vi "13-14-高级计算器.vi"() -> ()   [LabVIEW 2025]
panel:
  out "过程显示":string
  in  "清除":bool
  in  "等于":bool
  in  "小数点":bool
  in  "±号":bool
  in  "数字0":bool
  in  "操作/":bool
  in  "操作*":bool
  in  "数字9":bool
  in  "数字8":bool
  in  "数字7":bool
  in  "数字6":bool
  in  "数字5":bool
  in  "数字4":bool
  in  "操作-":bool
  in  "操作+":bool
  in  "数字3":bool
  in  "数字2":bool
  in  "数字1":bool
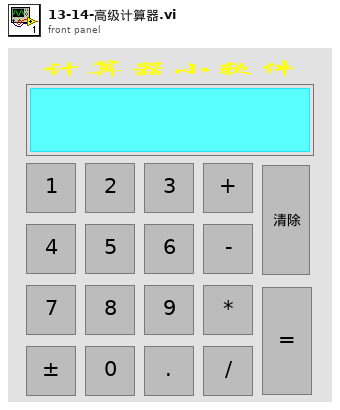
[diagram p1: front panel]
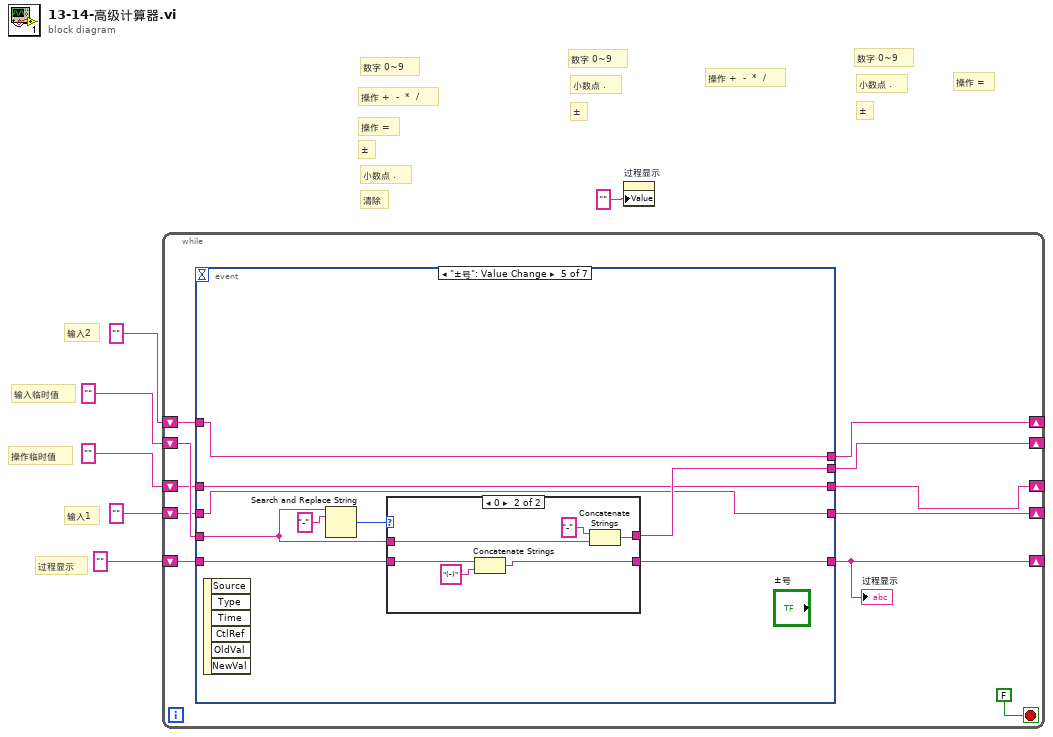
[diagram p0: block diagram]
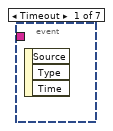
[diagram p2: hidden frame]
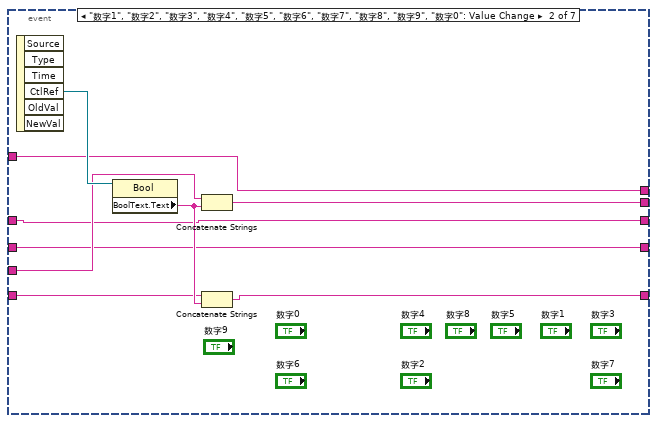
[diagram p3: hidden frame]
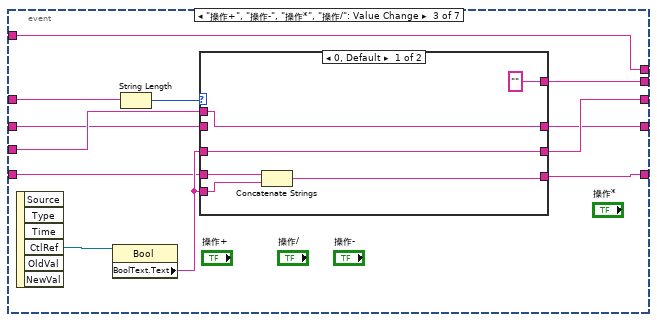
[diagram p4: hidden frame]
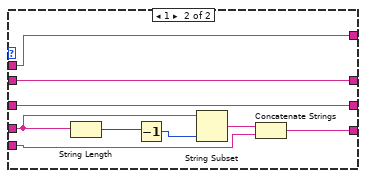
[diagram p5: hidden frame]
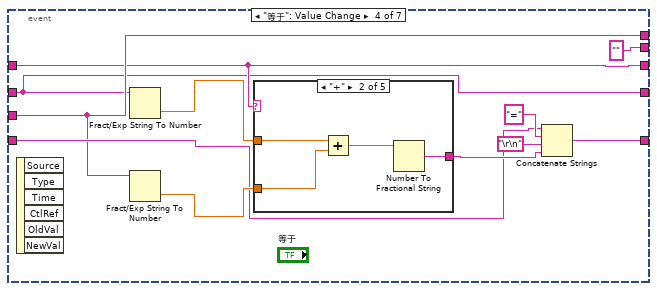
[diagram p6: hidden frame]
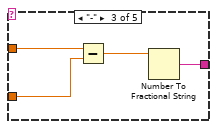
[diagram p8: hidden frame]
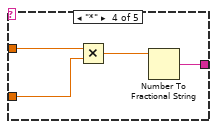
[diagram p9: hidden frame]
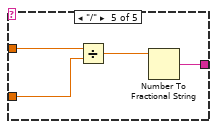
[diagram p10: hidden frame]
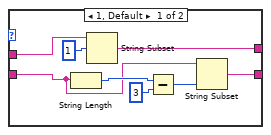
[diagram p11: hidden frame]
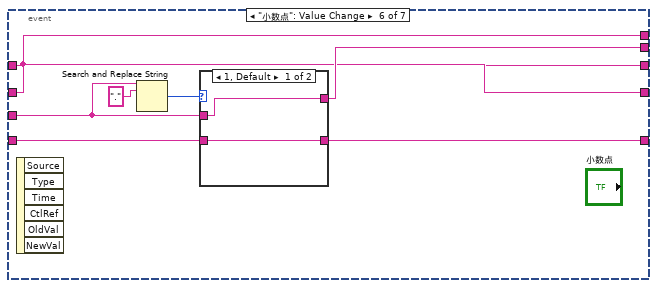
[diagram p12: hidden frame]
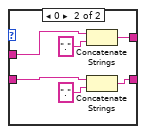
[diagram p13: hidden frame]
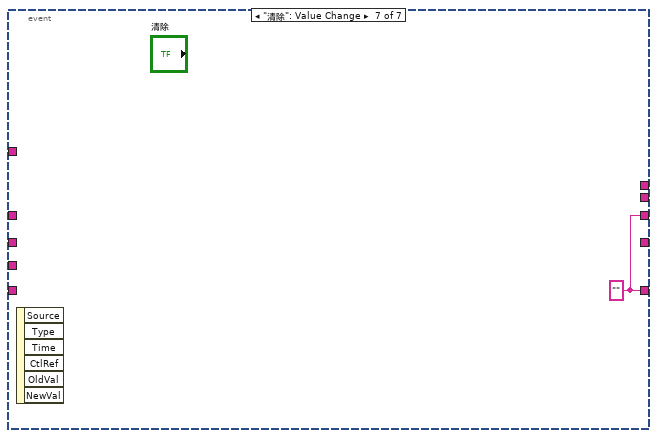
[diagram p14: hidden frame]
diagram:
  # "操作临时值"
  # "过程显示"
  # "输入2"
  # "输入1"
  # "输入临时值"
  # "操作 ="
  # "±"
  # "小数点 ."
  # "数字 0~9"
  # "操作 +  -  *  /"
  # "±"
  # "小数点 ."
  # "数字 0~9"
  # "清除"
  # "小数点 ."
  # "±"
  # "操作 ="
  # "操作 +  -  *  /"
  # "数字 0~9"
  n1 = while {
    shift-right: [w15] -> _
    shift-left: "" ("输入1") -> [w16]
    shift-right: [w11] -> _
    shift-left: "" ("输入1") -> [w10]
    shift-right: [w9] -> _
    shift-left: "" ("输入1") -> [w8]
    shift-right: [w7] -> _
    shift-left: "" ("输入1") -> [w14]
    shift-right: [w12] -> _
    shift-left: "" ("输入1") -> [w13]
    stop <- FALSE stop-if-true
    n2 = event shown="[4] \"±号\": Value Change" {
      selector: _ -> [_ _ _ _ _ _ _]
      dyn-events: _ -> [_ _ _ _ _ _ _]
      timeout: _ -> [_ _ _ _ _ _ _]
      tunnel: w16 -> [_ w24 w32 w56 w85 w109 _]
      tunnel: [_ w23 w30 "" ("输入临时值") w84 w108 _] -> w15
      tunnel: w14 -> [_ w22 w35 w59 w87 w107 _]
      tunnel: [_ w21 w34 w58 w86 w106 w120] -> w7
      tunnel: w13 -> [_ w18 w28 w55 w83 w104 _]
      tunnel: [_ w18 w33 w55 w83 w104 w120] -> w12
      tunnel: [_ w20 w31 w54 w82 w105 _] -> w11
      tunnel: w10 -> [_ w20 w29 w54 w82 w105 _]
      tunnel: [_ w19 w27 w56 w81 w105 _] -> w9
      tunnel: w8 -> [_ w19 w27 _ w81 _ _]
      event Timeout {
        n3 = event-data() -> ()  [unwired: 1 in, 3 out]
      }
      event "数字1", "数字2", "数字3", "数字4", "数字5", "数字6", "数字7", "数字8", "数字9", "数字0": Value Change {
        n4 = event-data() -> ("CtlRef"=w26:refnum<vi>)  [unwired: 1 in, 5 out]
        n5 = property class="Bool"(reference=w26) -> ("BoolText.Text"=w25:string)  [unwired: 1 in, 2 out]
        n6 = Concatenate Strings(w24, w25) -> (w23:string)
        n7 = Concatenate Strings(w22, w25) -> (w21:string)
      }
      event "操作+", "操作-", "操作*", "操作/": Value Change {
        n8 = event-data() -> ("CtlRef"=w38:refnum<vi>)  [unwired: 1 in, 5 out]
        n9 = property class="Bool"(reference=w38) -> ("BoolText.Text"=w36:string)  [unwired: 1 in, 2 out]
        n10 = String Length(string=w28) -> (length=w37:i32)
        n11 = case shown="0, Default" w37 {
          tunnel: w36 -> [w41 w47]
          tunnel: w36 -> [w44 w50]
          tunnel: w35 -> [w43 w49]
          tunnel: [w42 w48] -> w34
          tunnel: [w41 w47] -> w33
          tunnel: w32 -> [w40 w45]
          tunnel: [w40 w46] -> w31
          tunnel: ["" ("输入临时值") w45] -> w30
          tunnel: w29 -> [_ w46]
          frame 0, Default {
            n12 = Concatenate Strings(w43, w44) -> (w42:string)
          }
          frame 1 {
            n13 = String Length(string=w49) -> (length=w53:i32)
            n14 = Decrement(x=w53) -> (x-1=w52:i32)
            n15 = String Subset(string=w49, length (rest)=w52) -> (substring=w51:string)  [unwired: 1 in]
            n16 = Concatenate Strings(w51, w50) -> (w48:string)
          }
        }
      }
      event "等于": Value Change {
        n17 = event-data() -> ()  [unwired: 1 in, 6 out]
        n18 = Fract/Exp String To Number(string=w54) -> (number=w64:dbl)  [unwired: 3 in, 1 out]
        n19 = Fract/Exp String To Number(string=w56) -> (number=w63:dbl)  [unwired: 3 in, 1 out]
        n20 = case shown="\"+\"" w55 {
          tunnel: w64 -> [_ w68 w71 w75 w79]
          tunnel: w63 -> [_ w67 w70 w74 w80]
          tunnel: [_ w65 w69 w73 w78] -> w60
          frame "假", Default {
          }
          frame "+" {
            n21 = Add(x=w68, y=w67) -> (x+y=w66:dbl)
            n22 = Number To Fractional String(number=w66) -> (F-format string=w65:string)  [unwired: 3 in]
          }
          frame "-" {
            n23 = Subtract(x=w71, y=w70) -> (x-y=w72:dbl)
            n24 = Number To Fractional String(number=w72) -> (F-format string=w69:string)  [unwired: 3 in]
          }
          frame "*" {
            n25 = Multiply(x=w75, y=w74) -> (x*y=w76:dbl)
            n26 = Number To Fractional String(number=w76) -> (F-format string=w73:string)  [unwired: 3 in]
          }
          frame "/" {
            n27 = Divide(x=w79, y=w80) -> (x/y=w77:dbl)
            n28 = Number To Fractional String(number=w77) -> (F-format string=w78:string)  [unwired: 3 in]
          }
        }
        n29 = Concatenate Strings(w59, "=" ("字符串"), "\r\n", w60) -> (w58:string)
      }
      event "±号": Value Change {
        n30 = event-data() -> ()  [unwired: 1 in, 6 out]
        n31 = Search and Replace String(input string=w85, search string="-" ("搜索字符串")) -> (number of replacements=w88:i32)  [unwired: 6 in, 3 out]
        n32 = case shown="0" w88 {
          tunnel: w87 -> [w93 w101]
          tunnel: [w92 w100] -> w86
          tunnel: w85 -> [w91 w99]
          tunnel: [w90 w98] -> w84
          frame 1, Default {
            n33 = String Length(string=w93) -> (length=w96:i32)
            n34 = String Subset(string=w91, offset (0)=1 ("偏移量(0)")) -> (substring=w90:string)  [unwired: 1 in]
            n35 = Subtract(x=w96, y=3) -> (x-y=w94:i32)
            n36 = String Subset(string=w93, length (rest)=w94) -> (substring=w92:string)  [unwired: 1 in]
          }
          frame 0 {
            n37 = Concatenate Strings(w101, "(-)" ("字符串")) -> (w100:string)
            n38 = Concatenate Strings("-" ("字符串"), w99) -> (w98:string)
          }
        }
      }
      event "小数点": Value Change {
        n39 = event-data() -> ()  [unwired: 1 in, 6 out]
        n40 = Search and Replace String(input string=w109, search string="." ("搜索字符串")) -> (number of replacements=w110:i32)  [unwired: 6 in, 3 out]
        n41 = case shown="1, Default" w110 {
          tunnel: w109 -> [w113 w117]
          tunnel: [w113 w116] -> w108
          tunnel: w107 -> [w112 w115]
          tunnel: [w112 w114] -> w106
          frame 1, Default {
          }
          frame 0 {
            n42 = Concatenate Strings(w117, "." ("字符串")) -> (w116:string)
            n43 = Concatenate Strings(w115, "." ("字符串")) -> (w114:string)
          }
        }
      }
      event "清除": Value Change {
        w120 = "" ("操作临时值")
        n44 = event-data() -> ()  [unwired: 1 in, 6 out]
      }
    }
    "过程显示" <- w7
  }
  n45 = property on="过程显示" class="Str"("Value"="" ("过程显示")) -> ()  [unwired: 2 in, 2 out]
